vi "cube Immediate with Deadband.vi"(7 "Description":string, 8 "Command Info In":T1, 9 "Deadband Value":dbl=0.01, 10 "Conveyor Setpoint":dbl, 11 "Arm Setpoint":dbl) -> (0 "Command Info Out":T1)   [LabVIEW 2018]
doc: "This template includes code for deadband comparision to avoid excessive command scheduling. It is particularly useful for joystick-driven commands.\n\nBe sure to right-click and select New from Template and save with a new command name."
uses:
  <vilib>/Rock Robotics/WPI/Framework/Command Status Info.ctl
  <vilib>/Rock Robotics/WPI/Framework/Completion Status.ctl
  <vilib>/Rock Robotics/WPI/Framework/Completion Notifier.ctl
  Implementation/cube Setpoints.ctl
  Implementation/cube Operations.ctl
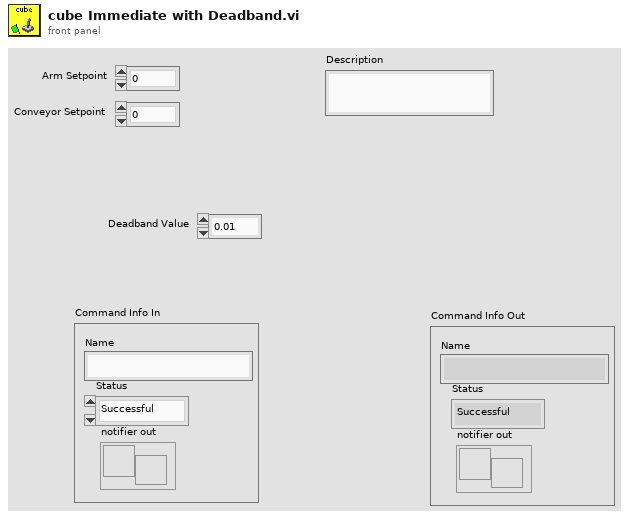
[diagram p1: front panel]
types:
  T1 = typedef "Command Status Info.ctl" = cluster{"Name":string, "Status":T2, "notifier out":T3}
  T2 = typedef "Completion Status.ctl" = enum16{"Successful", "Aborted", "Incomplete"}
  T3 = typedef "Completion Notifier.ctl" = refnum<notifier>
  T4 = typedef "cube Setpoints.ctl" = cluster{"Operation":T5, "Arm Setpoint":dbl, "Duration":dbl, "Conveyor Setpoint":dbl}
  T5 = typedef "cube Operations.ctl" = enum16{"Reserve", "Read Current", "Immediate", "Chew", "Puke", "Swallow", "Poop", "SpitFast", "SpitSlow"}
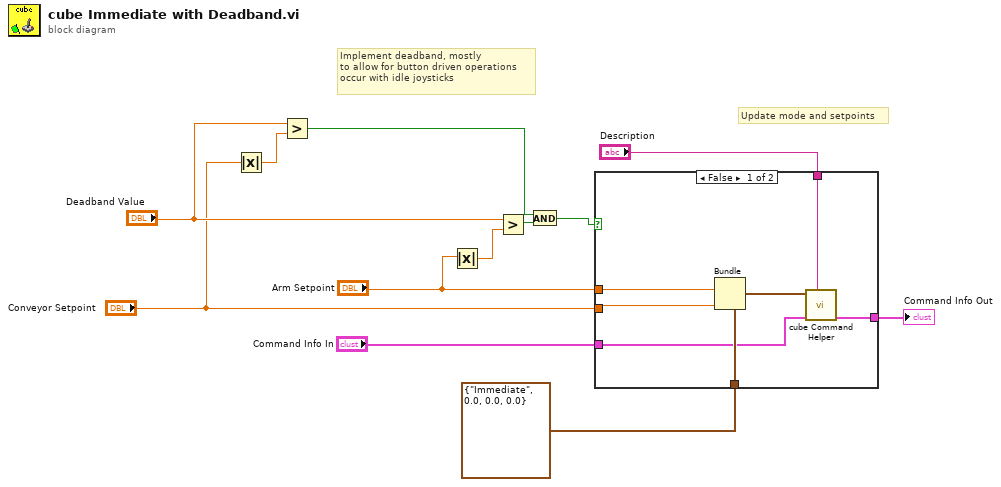
[diagram p0: block diagram]
diagram:
  # "Implement deadband, mostly\nto allow for button driven operations\noccur with idle joysticks"
  # "Update mode and setpoints"
  n1 = Absolute Value(x="Conveyor Setpoint") -> (abs(x)=w6:dbl)
  n2 = Greater?(x="Deadband Value", y=w6) -> (0:w2:bool)
  n3 = Absolute Value(x="Arm Setpoint") -> (abs(x)=w12:dbl)
  n4 = Greater?(x="Deadband Value", y=w12) -> (0:w3:bool)
  n5 = And(x=w2, y=w3) -> (x .and. y?=w4:bool)
  n6 = case shown="False" w4 {
    tunnel: "Arm Setpoint" -> [w19 _]
    tunnel: T4 {"Operation"=enum."Immediate", "Arm Setpoint"=0.0, "Duration"=0.0, "Conveyor Setpoint"=0.0} ("SubSystem Data") -> [w18 _]
    tunnel: [w17 w20] -> w11
    tunnel: "Command Info In" -> [w16 w20]
    tunnel: "Description" -> [w14 _]
    tunnel: "Conveyor Setpoint" -> [w13 _]
    frame False {
      n7 = Bundle(cluster=w18, "Arm Setpoint"=w19, "Conveyor Setpoint"=w13) -> (w15:T4)  [unwired: 2 in]
      n8 = call "cube Command Helper.vi"("Description"=w14, "Command Info In"=w16, "SubSystem Data"=w15) -> ("Command Info Out"=w17:T1)  [unwired: 6 in, 2 out]
    }
    frame True {
    }
  }
  "Command Info Out" <- w11
